vi "Valve_Init.vi"(0 "object in":refnum<class "Valve.lvclass">, 2 "VISA resource name":refnum<visa-resource-name>, 5 "error in (no error)":errorcluster) -> (14 "object out":refnum<class "Valve.lvclass">, 19 "error out":errorcluster)   [LabVIEW 2019, in "Valve.lvclass"]
uses:
  Valve.lvclass
  Valve.lvclass/Valve.ctl
  <vilib>/Instr/_visa.llb/VISA Configure Serial Port (Instr).vi
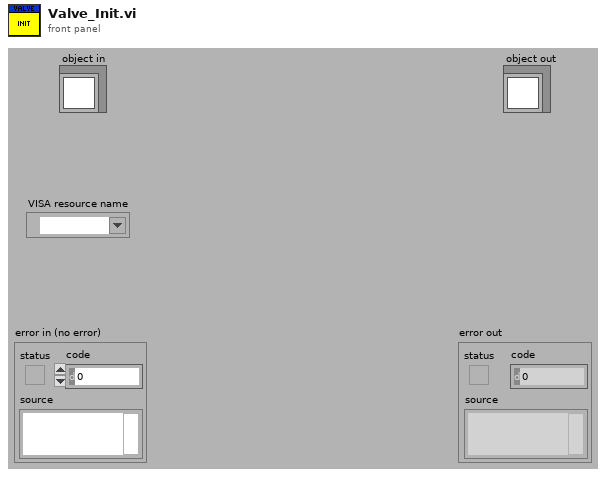
[diagram p1: front panel]
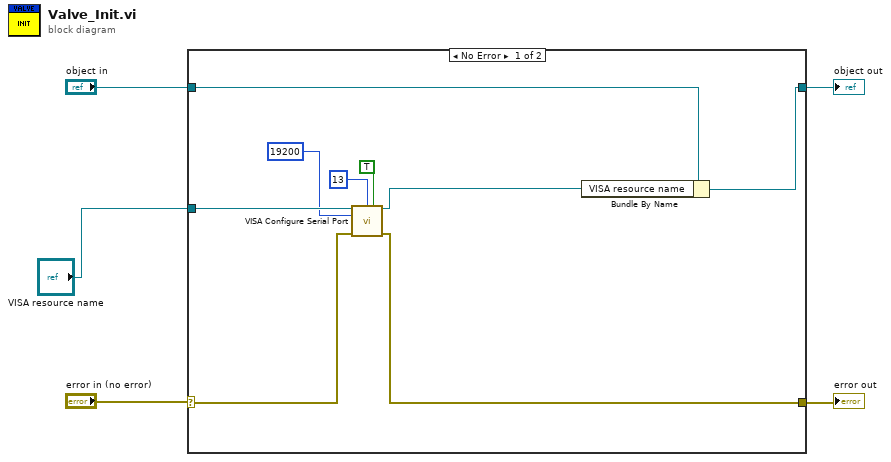
[diagram p0: block diagram]
diagram:
  n1 = case shown="No Error" "error in (no error)" {
    selector: "error in (no error)" -> [w12 w15]
    tunnel: "object in" -> [w14 w16]
    tunnel: [w13 w16] -> w4
    tunnel: [w7 w15] -> w2
    tunnel: "VISA resource name" -> [w10 _]
    frame No Error {
      n2 = call-poly "VISA Configure Serial Port"("VISA resource name"=w10, "termination char\n(0xA = '\\n' = LF)"=u8 13 ("termination char\n(0xA = '\\n' = LF)"), "Enable Termination\nChar (T)"=TRUE ("Enable Termination\nChar (T)"), "baud rate (9600)"=u32 19200, "error in (no error)"=w12) -> ("VISA resource name out"=w6:refnum<visa-resource-name>, "error out"=w7:errorcluster)  [unwired: 9 in]
      n3 = Bundle By Name(cluster=w14, "VISA resource name"=w6) -> (w13:refnum<class "Valve.lvclass">)
    }
    frame Error {
    }
  }
  "object out" <- w4
  "error out" <- w2
